vi "Set Initial Halt Button.vi"(8 "error in (no error)":errorcluster, 10 "Digital Inputs":T1, 11 "GripsMaster in":refnum<class "GripsMaster.lvclass">) -> (0 "error out":errorcluster, 3 "GripsMaster out":refnum<class "GripsMaster.lvclass">)   [LabVIEW 2013, in "GripsMaster.lvclass"]
uses:
  GripsMaster.lvclass
  controls/Digital Values.ctl
  GripsMaster.lvclass/GripsMaster.ctl
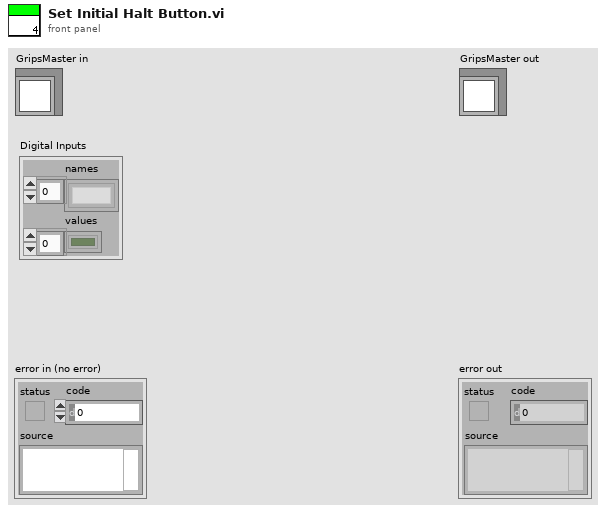
[diagram p1: front panel]
types:
  T1 = typedef "Digital Values.ctl" = cluster{"names":string[], "values":bool[]}
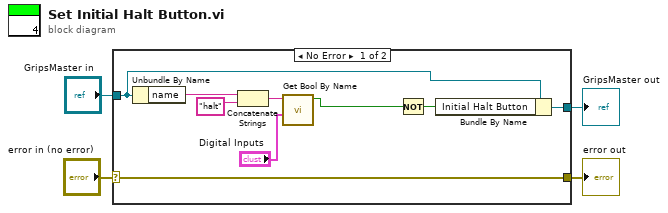
[diagram p0: block diagram]
diagram:
  n1 = case shown="No Error" "error in (no error)" {
    selector: "error in (no error)" -> [w13 w15]
    tunnel: [w13 w15] -> w3
    tunnel: [w12 w14] -> w1
    tunnel: "GripsMaster in" -> [w10 w14]
    frame No Error {
      n2 = Unbundle By Name(w10) -> ("name"=w9:string)
      n3 = Concatenate Strings(w9, "halt" ("y")) -> (w8:string)
      n4 = call "Get Bool By Name.vi"("name"=w8, "Digital Values"="Digital Inputs") -> ("result"=w6:bool)  [unwired: 7 in, 1 out]
      n5 = Not(x=w6) -> (.not. x?=w7:bool)
      n6 = Bundle By Name(cluster=w10, "Initial Halt Button"=w7) -> (w12:refnum<class "GripsMaster.lvclass">)
    }
    frame Error {
    }
  }
  "error out" <- w3
  "GripsMaster out" <- w1
